vi "Actor Core.vi"(8 "error in":errorcluster, 11 "Common in":refnum<class "Common.lvclass">) -> (0 "error out":errorcluster, 3 "Actor out":refnum<class "Actor.lvclass">)   [LabVIEW 2021, in "Common.lvlib" / "Common.lvclass"]
doc: "(<B>Filename</B>: Actor Framework.lvlib:Actor.lvclass:Actor Core.vi)\n\nReceives messages to the actor, reacts to them, and initiates any error handling that may shut the actor down.\n\nDescendant classes may override this VI to append parallel tasks for the actor to complete while it handles messages. Overrides use the Call Parent Class Method node."
uses:
  Common.lvclass
  C:/Program Files (x86)/National Instruments/LabVIEW 2021/vi.lib/ActorFramework/Actor/Actor.lvclass
  <vilib>/ActorFramework/Actor/Actor.lvclass
  <vilib>/ActorFramework/Actor/Actor.lvclass/Actor.ctl
  <vilib>/ActorFramework/Message Enqueuer/Message Enqueuer.lvclass/Message Enqueuer.ctl
  Common.lvclass/Common.ctl
  <vilib>/ActorFramework/Message Enqueuer/Init from Existing Queue.vi
  <vilib>/ActorFramework/Message Enqueuer/Enqueue.vi
  <vilib>/ActorFramework/Stop Msg/Stop Msg.lvclass
  C:/Program Files (x86)/National Instruments/LabVIEW 2021/vi.lib/ActorFramework/Message/Message.lvclass
  <vilib>/ActorFramework/Message Priority Queue/Priority Enqueue.vi
  <vilib>/MGI/Monitored Actor/Monitored Actor/Monitored Actor/Monitored Actor.lvclass
  <vilib>/ActorFramework/Message Enqueuer/Message Enqueuer.lvclass
panel:
  out "messages":T1(array[cluster]) {"Time Stamp" format="%<%x %.3X>T"}
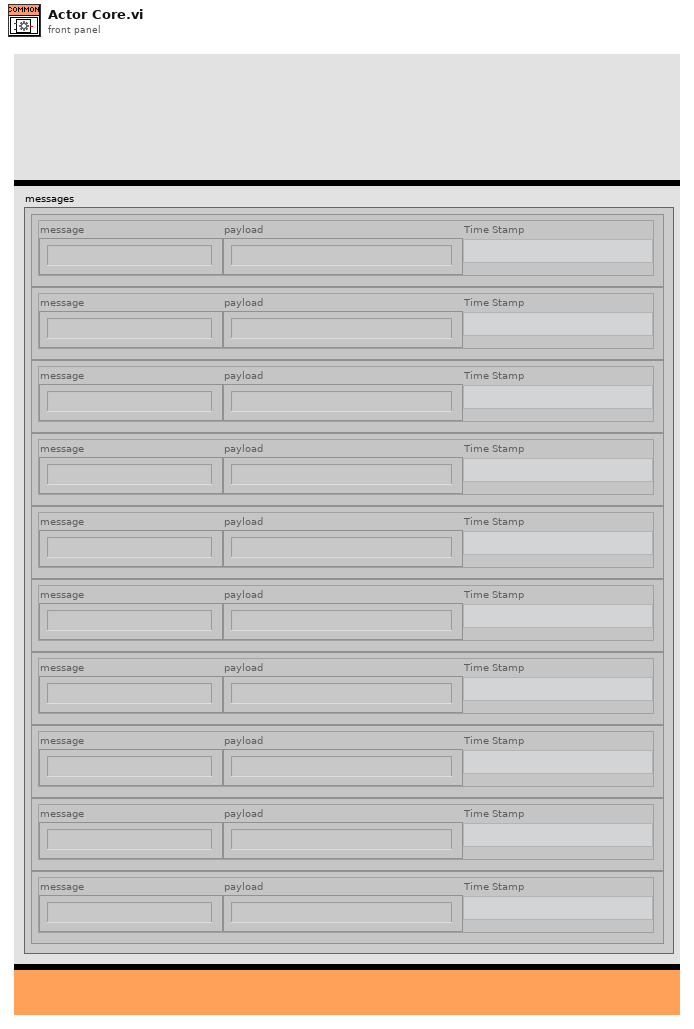
[diagram p1: front panel]
types:
  T1 = cluster{"message":string, "payload":string, "Time Stamp":timestamp}[]
  T2 = cluster{"Stop":refnum<user-event>, "message received":refnum<user-event>}
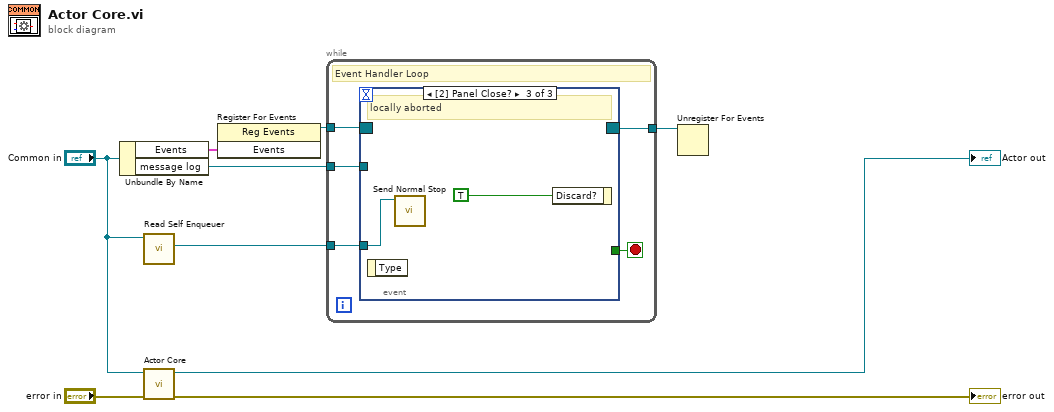
[diagram p0: block diagram]
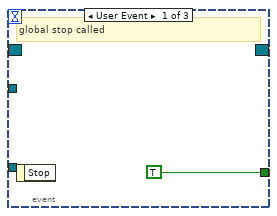
[diagram p2: hidden frame]
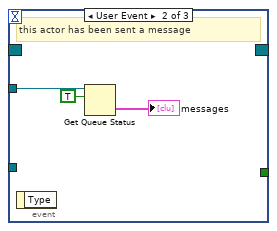
[diagram p3: hidden frame]
diagram:
  n1 = Unbundle By Name("Common in") -> ("Events"=w5:T2, "message log"=w1:refnum<queue>)
  n2 = call <vilib>:"Read Self Enqueuer.vi"("Actor"="Common in") -> ("Self Enqueuer"=w2:refnum<class "Message Enqueuer.lvclass">)  [unwired: 10 in]
  n3 = call-parent "Actor Core.vi"("error in"="error in", "Actor in"="Common in") -> ("error out"=→"error out":errorcluster, "Actor out"=→"Actor out":refnum<class "Actor.lvclass">)  [unwired: 8 in]
  n4 = register-events(w5) -> (reference out=w4:refnum<event-registration>)  [unwired: 2 in, 1 out]
  n5 = while {
    tunnel: w4 -> [w14]
    tunnel: [w12] -> w6
    tunnel: w2 -> [w11]
    tunnel: w1 -> [w10]
    stop <- w13 stop-if-true
    # "Event Handler Loop"
    n6 = event shown="[2] Panel Close?" {
      selector: w14 -> [_ _ _]
      dyn-events: [_ _ _] -> w12
      timeout: _ -> [_ _ _]
      tunnel: [TRUE _ _] -> w13
      tunnel: w11 -> [_ _ w19]
      tunnel: w10 -> [_ w18 _]
      event User Event {
        # "global stop called"
        n7 = event-data() -> ()  [unwired: 1 in, 1 out]
      }
      event User Event {
        # "this actor has been sent a message"
        n8 = event-data() -> ()  [unwired: 1 in, 1 out]
        n9 = Get Queue Status(queue=w18, return elements? (F)=TRUE) -> (elements=→"messages":T1)  [unwired: 1 in, 7 out]
      }
      event Panel Close? {
        # "locally aborted"
        n10 = event-data() -> ()  [unwired: 1 in, 1 out]
        n11 = call <vilib>:"Send Normal Stop.vi"("Message Enqueuer"=w19) -> ()  [unwired: 10 in, 1 out]
        n12 = event-data("Discard?"=TRUE) -> ()  [unwired: 1 in, 1 out]
      }
    }
  }
  n13 = Unregister For Events(event registration refnum=w6) -> ()  [unwired: 1 in, 1 out]
